vi "OpenAngleToGoal.vi"(5 "Ally?":bool, 7 "Gap Coord":dbl[](array[numeric]), 8 "error in (no error)":errorcluster, 9 "Game":refnum<class "Game.lvclass">, 10 "Point":dbl[](array[numeric]), 11 "object in":refnum<class "Utilities.lvclass">) -> (0 "error out":errorcluster, 2 "Evaluation":dbl, 3 "object out":refnum<class "Utilities.lvclass">)   [LabVIEW 2023, in "Utilities.lvclass"]
uses:
  Utilities.lvclass
  Game_class/Game.lvclass
  Game_class/Game.lvclass/Game.ctl
  Game_class/Read FieldRef.vi
  Game_class/Read NewParameters.vi
  Game_class/Read Utilities.lvclass.vi
  Field_class/Field.lvclass
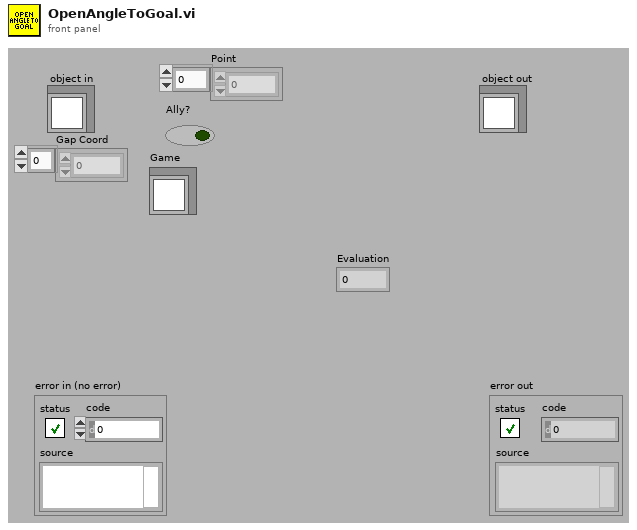
[diagram p1: front panel]
types:
  T1 = typedef "NewParameters.ctl" = cluster{"PenaltyDistance":dbl, "DistanceAttackerToBackBall":dbl, "Division":enum16{"Div B", "Div A"}, "DistanceToAvoidyEnemyRobot":dbl, "BallPlacementDistance":dbl, "DisatanceBehindBallToStealBall":dbl, "MaxDistanceToPositionKickoff":dbl, "BlockEnemyTarget":bool, "MaxStopVAng":dbl, "DistanceMarkerToEnemy":dbl, "IgnoreDribblerContact":bool, "DistanceToBeginEnemyPosession":dbl, "GoToBallWhenEnemyNotMoving":bool, "EnemyDistanceToReduceVelocity":dbl, "TurnOnEnemyDistanceToReduceVelocity":bool, "EnemyDistanceToShootOutBall":dbl, "DefenseKickBall":bool, "MoreKickToGoal? (0-0.3)":dbl, "ChipKickInEnemyField":bool, "ShootOutRobotId":dbl, "FieldLenghtDenominatorInShootOut":dbl, "AdjustPositionInBallPlacement":bool, "PowerGodPass":dbl, "VelocityAbortEnemyPos":dbl, "MaxDistToBeginPass":dbl, "MinDistToBeginPass":dbl, "VelocityInDirects":dbl, "BadDribblerIDs":i32[], "NewKickToDistanceAroundBall":dbl, "PowerAvoidColisionMarker":dbl, "DistanceToAvoidColisionMarker":dbl, "AvoidBallKick":dbl, "DistanceTryKick":dbl, "SuicideKickDIstance":dbl, "AdjustFirstKickDistance":dbl, "AvoidAimLessKick":dbl, "DistanceToAvoidyEnemyShootRobot ":dbl, "NumberOfMarkers":dbl, "PotField":bool, "PIDLateral":bool, "MinDistanceFirstKickX":dbl, "MinDistanceFirstKickY":dbl, "FractionOfDistToTouchGround\nAfterChipKick":dbl, "FractionOfKickxWhen\nComposedWithKickz":dbl, "Style":T2, "MoveInTurnState":bool, "DistFromEnemyToConsider\nMoveInTurnState":dbl, "CascadePID":bool, "TurnAroundParameters":cluster{"Radius":dbl, "Multiplier":dbl, "ChordAngle":dbl}, "SafeDriveVel":dbl, "DistanceToGoToBackBall":dbl, "minDistanceToNotFinishEnemyPossession":dbl, "OneTouchShot":cluster{"angleFactor":dbl, "maxAngle":dbl, "Attack":bool, "Defense":bool}, "OpenAngleToGoal":cluster{"minAngle":dbl, "maxAngle":dbl, "minEvaluation":dbl}, "ShotInterception":cluster{"shotSpeed":dbl, "minEnemySpeed":dbl, "maxEnemySpeed":dbl, "minEvaluation":dbl}, "AllyTeamArray":T3[], "maxDefendersNumber":i32, "Zone":cluster{"GuardPositionArray":dbl[][], "ZoneMidField":dbl[], "CenterForwardWidth":dbl}, "MinEvaluationToShoot":dbl, "PassInterception":cluster{"maxPassSpeed":dbl, "minPassSpeed":dbl, "minEnemySpeed":dbl, "chipPassDistance":dbl, "chipPassEvaluation":dbl, "minEvaluation":dbl, "maxEnemySpeed":dbl}, "PassDistance":cluster{"maxDistance":dbl, "minDistance":dbl}}
  T2 = typedef "Style.ctl" = enum16{"Insanity", "Offensive", "Defensive"}
  T3 = typedef "AllyTeam.ctl" = enum16{"Keeper", "Defender", "Attacker"}
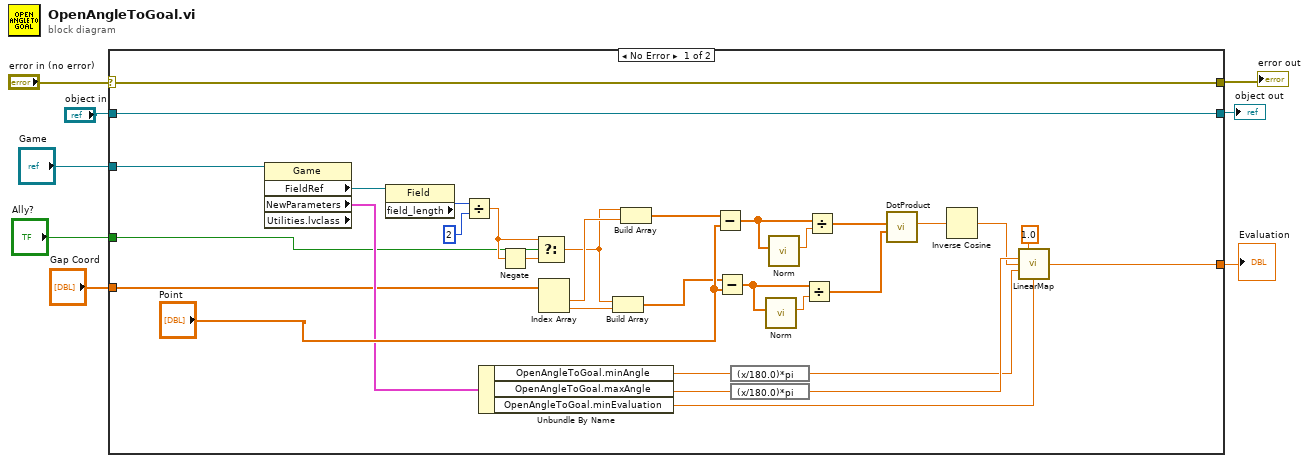
[diagram p0: block diagram]
diagram:
  n1 = case shown="No Error" "error in (no error)" {
    selector: "error in (no error)" -> [w40 w42]
    tunnel: [w40 w42] -> w7
    tunnel: [w39 w41] -> w5
    tunnel: "object in" -> [w39 w41]
    tunnel: "Game" -> [w19 _]
    tunnel: "Gap Coord" -> [w18 _]
    tunnel: [w17 _] -> w2
    tunnel: "Ally?" -> [w16 _]
    frame No Error {
      n2 = property class="Game" props=["FieldRef", "NewParameters", "Utilities.lvclass"](reference=w19) -> ("FieldRef"=w35:refnum<class "Field.lvclass">, "NewParameters"=w27:T1)  [unwired: 1 in, 3 out]
      n3 = property class="Field"(reference=w35) -> ("field_length"=w34:i32)  [unwired: 1 in, 2 out]
      n4 = Divide(x=w34, y=2) -> (x/y=w28:dbl)
      n5 = Unbundle By Name(w27) -> ("OpenAngleToGoal.minAngle"=w25:dbl, "OpenAngleToGoal.maxAngle"=w26:dbl, "OpenAngleToGoal.minEvaluation"=w21:dbl)
      n6 = Negate(x=w28) -> (-x=w29:dbl)
      n7 = Select(t=w28, s=w16, f=w29) -> (s? t:f=w30:dbl)
      n8 = Index Array(array=w18) -> (element #1=w37:dbl, element #2=w36:dbl)  [unwired: 2 in]
      n9 = Build Array(w30, w36) -> (w31:dbl[])
      n10 = Build Array(w30, w37) -> (w32:dbl[])
      n11 = Subtract(x=w32, y="Point") -> (x-y=w12:dbl[])
      n12 = Subtract(x=w31, y="Point") -> (x-y=w10:dbl[])
      n13 = expression code="(x/180.0)*pi" ("degrees to radians")(w25) -> (w22:dbl)
      n14 = expression code="(x/180.0)*pi" ("degrees to radians")(w26) -> (w24:dbl)
      n15 = call "Norm.vi"("2D vector"=w10) -> ("Modulo"=w9:dbl)  [unwired: 8 in, 2 out]
      n16 = call "Norm.vi"("2D vector"=w12) -> ("Modulo"=w11:dbl)  [unwired: 8 in, 2 out]
      n17 = Divide(x=w10, y=w9) -> (x/y=w14:dbl[])
      n18 = Divide(x=w12, y=w11) -> (x/y=w15:dbl[])
      n19 = call "DotProduct.vi"("Point2"=w14, "Point1"=w15) -> ("dot product"=w13:dbl)  [unwired: 7 in, 2 out]
      n20 = Inverse Cosine(1:w13) -> (0:w23:dbl)
      n21 = call "LinearMap.vi"("MaxY"=1.0 ("MaxEvalutation"), "MaxX"=w24, "X"=w23, "MinX"=w22, "MinY"=w21) -> ("Y"=w17:dbl)  [unwired: 8 in, 2 out]
    }
    frame Error {
    }
  }
  "error out" <- w7
  "object out" <- w5
  "Evaluation" <- w2
